vi "Start PJVS.vi"(6 "Requiested PJVS steps":u32, 7 "Requested PJVS frequency (Hz)":dbl, 8 "error in (pass through)":errorcluster, 10 "Maximal signal amplitude (V)":dbl, 11 "PJVS setup":T1={"PJVS type"=enum."AC-supraVOLTcontrol", "Status Refnum"=refnum, "AC-supraVOLTcontrol"={"IP address:port (0.0.0.0:0000)"="0.0.0.0:0000", "Timeouts"={"TCP Read & Write (ms)"=7000, "Sensors readout"=5000, "PJVS setup"=10000, "Nullmeter readout"=5000, "Multiplexer setup"=3000, "57XX setup"=15000, "Generator setup"=5000, "Synthesizer setup"=3000, "Sampler readout"=10000}, "Simulation mode"=FALSE, "Debug mode"=FALSE}, "NPL bias source"={"DataSocketCluster"={"Server Machine"="CZC", "Client Machine"="localhost", "Data"="P2", "TimeStamp"=0.0, "Count"=1, "Target Process"="General Server"}}, "Manual PJVS"={"PJVS frequency (Hz)"=0.0, "Reference voltages (V)"=[], "File with PJVS voltages"=path ""}, "VTT PJVS"={"some VTT only property"=""}} {"NPL bias source"."DataSocketCluster"."TimeStamp" format="%.2f"}) -> (0 "error out":errorcluster, 2 "PJVS reference voltages (1 period, V)":dbl[](array[numeric]), 3 "PJVS setup out":T1={"PJVS type"=enum."AC-supraVOLTcontrol", "Status Refnum"=refnum, "AC-supraVOLTcontrol"={"IP address:port (0.0.0.0:0000)"="0.0.0.0:0000", "Timeouts"={"TCP Read & Write (ms)"=7000, "Sensors readout"=5000, "PJVS setup"=10000, "Nullmeter readout"=5000, "Multiplexer setup"=3000, "57XX setup"=15000, "Generator setup"=5000, "Synthesizer setup"=3000, "Sampler readout"=10000}, "Simulation mode"=FALSE, "Debug mode"=FALSE}, "NPL bias source"={"DataSocketCluster"={"Server Machine"="CZC", "Client Machine"="localhost", "Data"="P2", "TimeStamp"=0.0, "Count"=1, "Target Process"="General Server"}}, "Manual PJVS"={"PJVS frequency (Hz)"=0.0, "Reference voltages (V)"=[], "File with PJVS voltages"=path ""}, "VTT PJVS"={"some VTT only property"=""}} {"NPL bias source"."DataSocketCluster"."TimeStamp" format="%.2f"}, 4 "Set PJVS steps":u32, 5 "Set frequency (Hz)":dbl)   [LabVIEW 2020]
doc: "Initialize the PJVS. Calls the initialization routine of the actual driver."
uses:
  Type definitions/PJVS.ctl
  Type definitions/PJVS Type.ctl
  external libraries/acsvcontrol-driver/Public/Type Definitions/Timeouts.ctl
  external libraries/JV modified NPL Bias source/DataSocketCluster external.ctl
  external libraries/acsvcontrol-driver/Public/Type Definitions/Waveform.ctl
  external libraries/acsvcontrol-driver/Public/Type Definitions/Multiplexer.ctl
  <vilib>/Utility/error.llb/Error Cluster From Error Code.vi
  <vilib>/ErrorRing/Error Ring.xnode
  external libraries/acsvcontrol-driver/ACSVcontrol-driver.lvlib
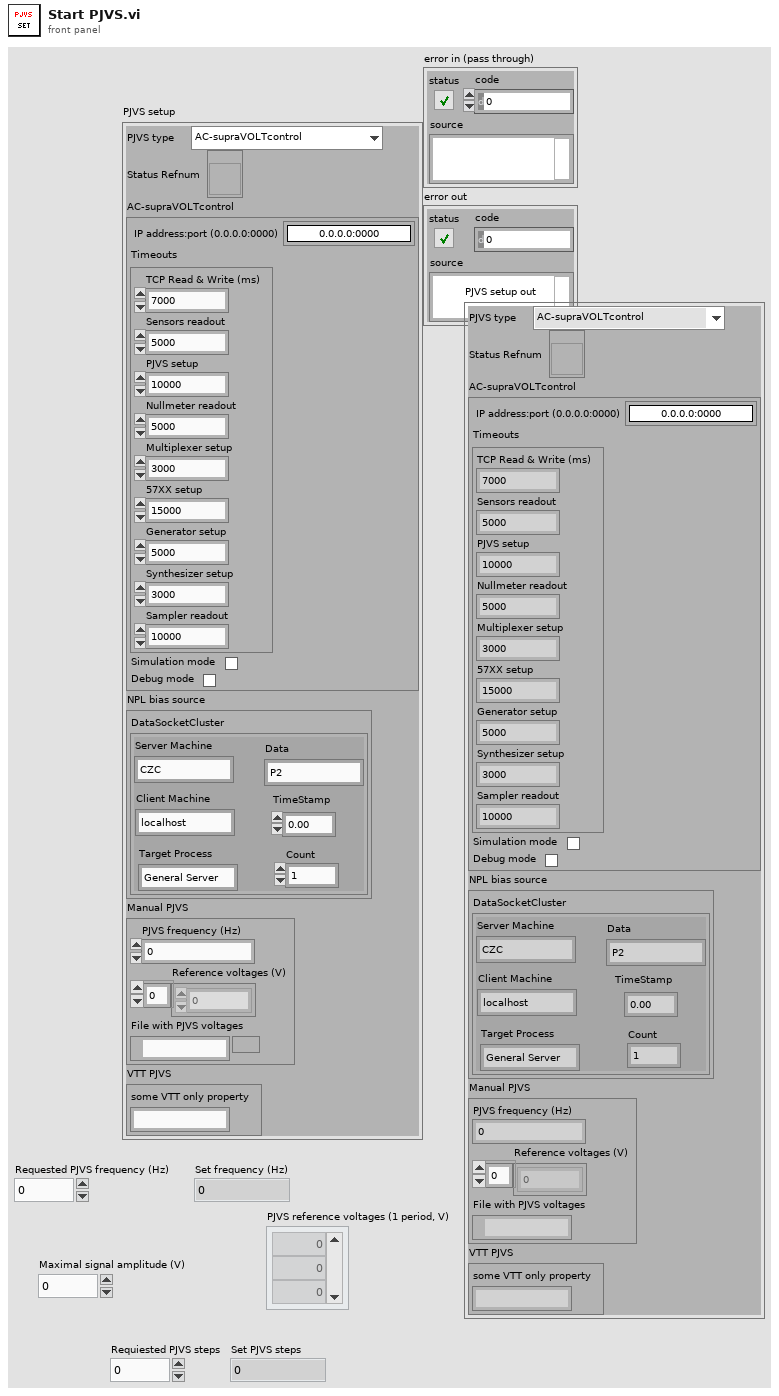
[diagram p1: front panel]
types:
  T1 = typedef "PJVS.ctl" = cluster{"PJVS type":T2, "Status Refnum":refnum<vi>, "AC-supraVOLTcontrol":cluster{"IP address:port (0.0.0.0:0000)":string, "Timeouts":T3, "Simulation mode":bool, "Debug mode":bool}, "NPL bias source":cluster{"DataSocketCluster":T4}, "Manual PJVS":cluster{"PJVS frequency (Hz)":dbl, "Reference voltages (V)":dbl[], "File with PJVS voltages":path}, "VTT PJVS":cluster{"some VTT only property":string}}
  T2 = typedef "PJVS Type.ctl" = enum16{"AC-supraVOLTcontrol", "JV modified NPL bias control", "Manual PJVS", "VTT PJVS"}
  T3 = typedef "ACSVcontrol-driver.lvlib/Timeouts.ctl" = cluster{"TCP Read & Write (ms)":i32, "Sensors readout":i32, "PJVS setup":i32, "Nullmeter readout":i32, "Multiplexer setup":i32, "57XX setup":i32, "Generator setup":i32, "Synthesizer setup":i32, "Sampler readout":i32}
  T4 = typedef "DataSocketCluster external.ctl" = cluster{"Server Machine":string, "Client Machine":string, "Data":string, "TimeStamp":dbl, "Count":i32, "Target Process":string}
  T5 = typedef "ACSVcontrol-driver.lvlib/Multiplexer.ctl" = enum16{"Short DC Nano / Voltmeter", "Short AC Sampler", "Short Switch DC (JVS->Nano)", "Short Switch AC (JVS->Digit)", "JVS-Voltmeter", "Channel A positive", "Channel A negative", "Channel B positive", "Channel B negative", "Channel C positive", "Channel C negative", "Nulldetector-Channel A+", "Nulldetector-Channel A-", "Nulldetector-Channel B+", "Nulldetector-Channel B-", "Nulldetector-Channel C+", "Nulldetector-Channel C-", "ext.Voltmeter-Channel A+", "ext.Voltmeter-Channel A-", "ext.Voltmeter-Channel B+", "ext.Voltmeter-Channel B-", "ext.Voltmeter-Channel C+", "ext.Voltmeter-Channel C-"}
  T6 = typedef "ACSVcontrol-driver.lvlib/Waveform.ctl" = enum16{"Sinewave", "Triangle", "Sawtooth", "Rectangle", "Arbitrary"}
  T7 = typedef "ACSVcontrol-driver.lvlib/PJVS Voltages.ctl" = cluster{"DC Voltage (S)":dbl, "AC Josephson Voltage RMS (V)":dbl, "Number of steps":i32, "AC Voltages (V)":dbl[]}
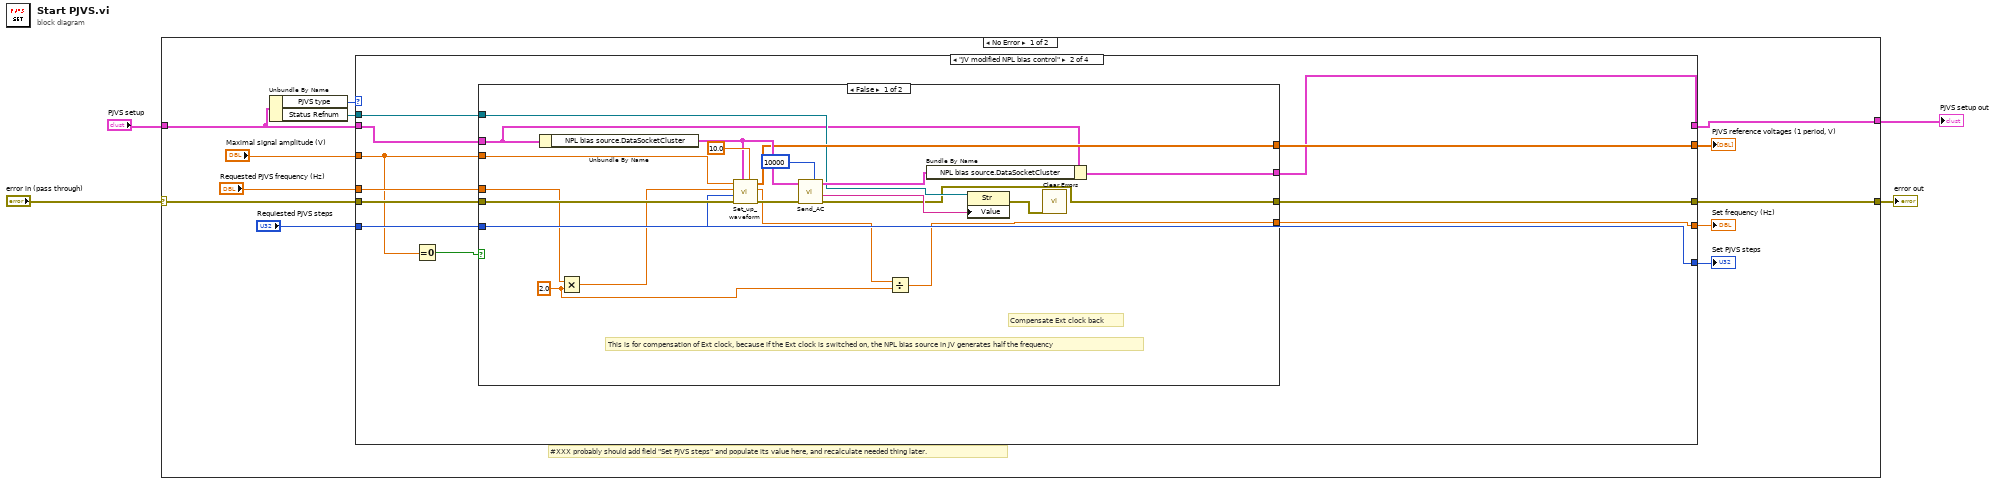
[diagram p0: block diagram]
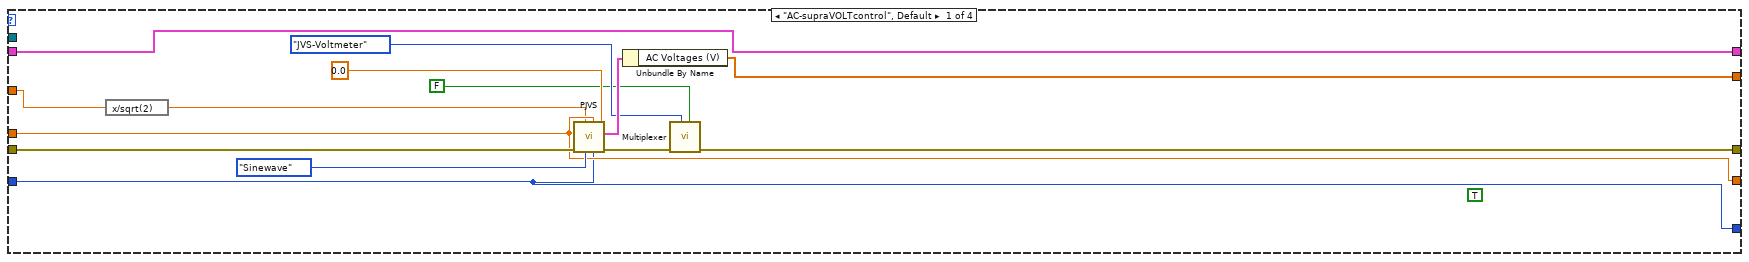
[diagram p2: hidden frame]
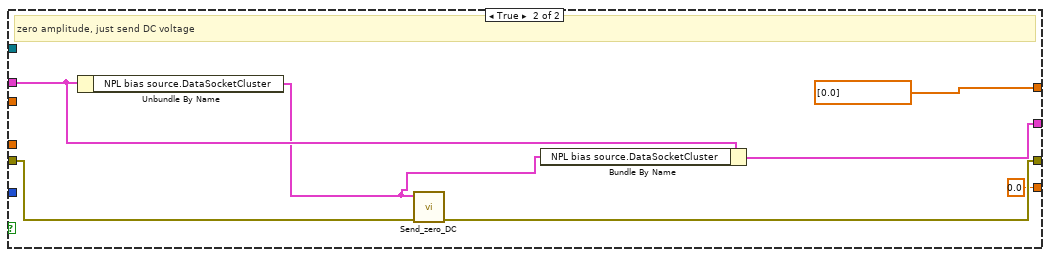
[diagram p3: hidden frame]
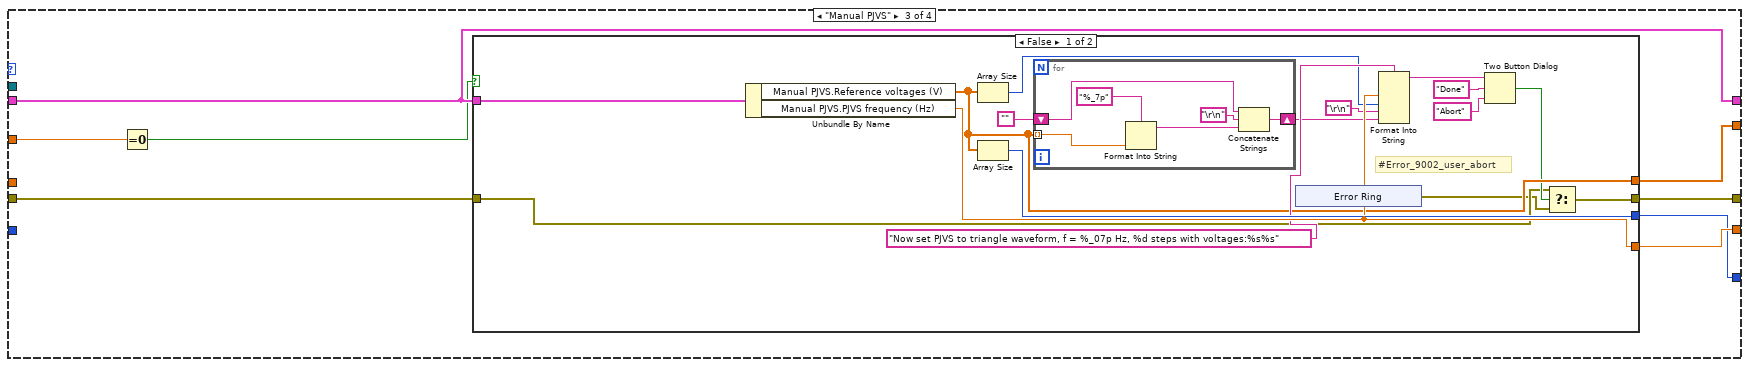
[diagram p4: hidden frame]
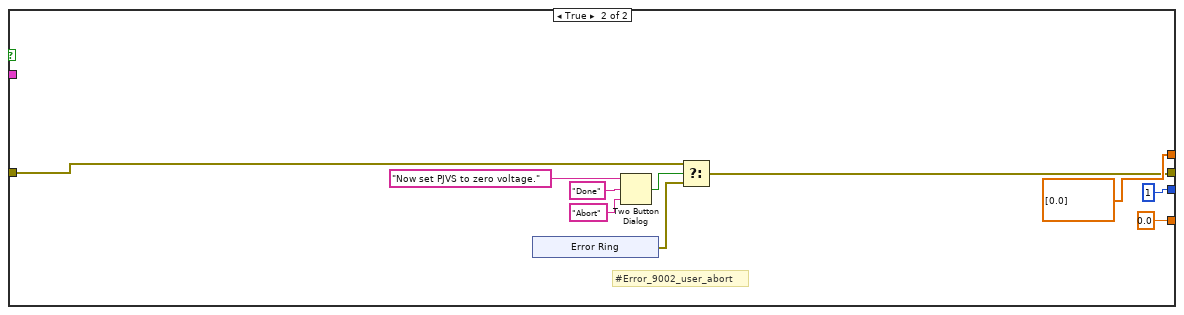
[diagram p5: hidden frame]
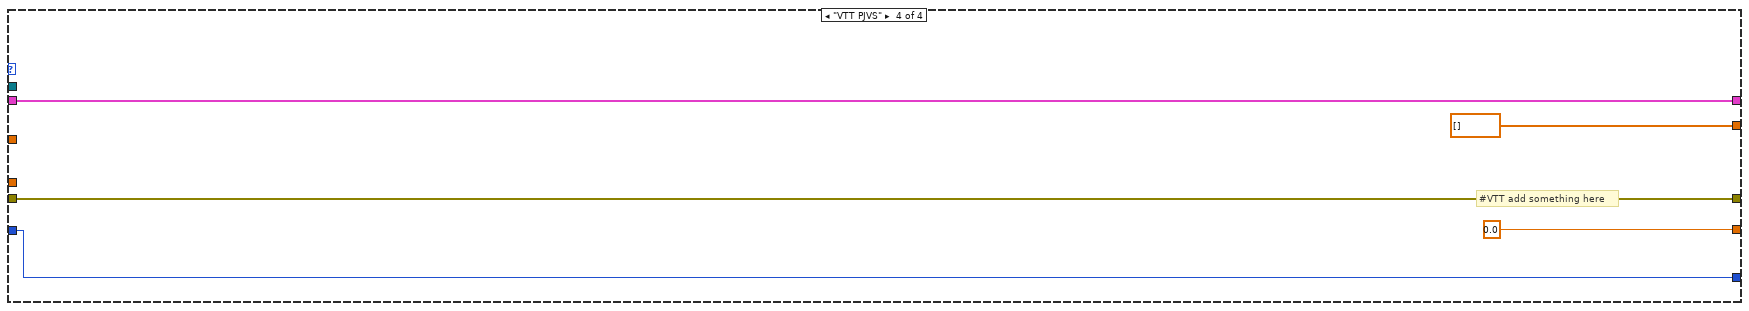
[diagram p6: hidden frame]
diagram:
  n1 = case shown="No Error" "error in (pass through)" {
    selector: "error in (pass through)" -> [w13 w125]
    tunnel: "PJVS setup" -> [w11 w124]
    tunnel: [w14 w125] -> w3
    tunnel: [w10 w124] -> w1
    frame No Error {
      # "#XXX probably should add field \"Set PJVS steps\" and populate its value here, and recalculate needed thing later."
      n2 = Unbundle By Name(w11) -> ("PJVS type"=w16:T2, "Status Refnum"=w15:refnum<vi>)
      n3 = case shown="\"JV modified NPL bias control\"" w16 {
        tunnel: w15 -> [_ w40 _ _]
        tunnel: w13 -> [w30 w39 w69 w122]
        tunnel: [w22 w38 w70 w122] -> w14
        tunnel: "Requested PJVS frequency (Hz)" -> [w21 w36 _ _]
        tunnel: "Maximal signal amplitude (V)" -> [w18 w34 w72 _]
        tunnel: "Requiested PJVS steps" -> [w19 w37 _ w119]
        tunnel: [w26 w41 w74 dbl[] [] ("Voltage at each step on PJVS curve")] -> w5
        tunnel: w11 -> [w20 w31 w76 w123]
        tunnel: [w21 w35 w75 0.0 ("Set frequency (Hz)")] -> w12
        tunnel: [w20 w32 w76 w123] -> w10
        tunnel: [w19 w37 w73 w119] -> w6
        frame "AC-supraVOLTcontrol", Default {
          (unwired) TRUE ("Waveform (F) (F:Sine, T:Square)")
          n4 = expression code="x/sqrt(2)"(w18) -> (w17:dbl)
          n5 = call "PJVS.vi"("Trim current (A) (+- 0.002)"=0.0, "Samples (2) (2 - 256)"=w19, "Frequency  (0 Hz) (0, 0.5 - 10e3)"=w21, "Waveform (Sinewave)"=Waveform."Sinewave", "Voltage (0 V DC/RMS) (DC: +- 10.1, AC: 0 - 7.2)"=w17, "error in (no error)"=w30) -> ("error out"=w25:errorcluster, "PJVS Voltages"=w27:T7)  [unwired: 4 in]
          n6 = Unbundle By Name(w27) -> ("AC Voltages (V)"=w26:dbl[])
          n7 = call "Multiplexer.vi"("AC (F) (F:Nano, T:Digitizer)"=FALSE, "Multiplexer (Short DC Nano / Voltmeter)"=Multiplexer."JVS-Voltmeter", "error in (no error)"=w25) -> ("error out"=w22:errorcluster)  [unwired: 8 in]
        }
        frame "JV modified NPL bias control" {
          n8 = Equal To 0?(x=w34) -> (x = 0?=w33:bool)
          n9 = case shown="False" w33 {
            tunnel: w34 -> [w59 _]
            tunnel: [w58 dbl[] [0.0] ("Voltage at each step on PJVS curve")] -> w41
            tunnel: w31 -> [w45 w68]
            tunnel: w40 -> [w55 _]
            tunnel: w39 -> [w53 w65]
            tunnel: [w43 w64] -> w38
            tunnel: w37 -> [w51 _]
            tunnel: w36 -> [w49 _]
            tunnel: [w46 0.0] -> w35
            tunnel: [w44 w67] -> w32
            frame False {
              w50 = 2.0 ("y")
              # "Compensate Ext clock back"
              # "This is for compensation of Ext clock, because if the Ext clock is switched on, the NPL bias source in JV generates half the frequency"
              n10 = Unbundle By Name(w45) -> ("NPL bias source.DataSocketCluster"=w60:T4)
              n11 = Multiply(x=w49, y=w50) -> (x*y=w48:dbl)
              n12 = call "Set_up_waveform.vi"("TimeOut Time (s)"=10.0, "DataSocketCluster In"=w60, "error in (no error)"=w53, "Steps on PJVS curve"=w51, "Frequency (Hz)"=w48, "Amplitude (V)"=w59) -> ("error IO"=w52:errorcluster, "Set frequency (Hz)"=w47:dbl, "Voltage at each step on PJVS curve"=w58:dbl[])  [unwired: 3 out]
              n13 = call "Send_AC.vi"("milliseconds to wait"=u32 10000, "error in (no error)"=w52, "DataSocketCluster In"=w60) -> ("error out"=w43:errorcluster, "Response to SEND AC"=w54:string, "DataSocketCluster out"=w56:T4)  [unwired: 6 in]
              n14 = Divide(x=w47, y=w50) -> (x/y=w46:dbl)
              n15 = Bundle By Name(cluster=w45, "NPL bias source.DataSocketCluster"=w56) -> (w44:T1)
              n16 = property class="Str"(reference=w55, "Value"=w54) -> (error out=w42:errorcluster)  [unwired: 1 in, 1 out]
              n17 = call <vilib>:"Clear Errors.vi"("error in (no error)"=w42) -> ()  [unwired: 5 in, 2 out]
            }
            frame True {
              # "zero amplitude, just send DC voltage"
              n18 = Unbundle By Name(w68) -> ("NPL bias source.DataSocketCluster"=w66:T4)
              n19 = call "Send_zero_DC.vi"("error in (no error)"=w65, "machine"=w66) -> ("error out"=w64:errorcluster)  [unwired: 8 in, 1 out]
              n20 = Bundle By Name(cluster=w68, "NPL bias source.DataSocketCluster"=w66) -> (w67:T1)
            }
          }
        }
        frame "Manual PJVS" {
          n21 = Equal To 0?(x=w72) -> (x = 0?=w71:bool)
          n22 = case shown="False" w71 {
            tunnel: w76 -> [w92 _]
            tunnel: [w90 0.0 ("PJVS frequency (Hz)")] -> w75
            tunnel: [w86 dbl[] [0.0] ("Reference voltages (V)")] -> w74
            tunnel: [w91 1] -> w73
            tunnel: w69 -> [w79 w106]
            tunnel: [w78 w105] -> w70
            frame False {
              # "#Error_9002_user_abort"
              n23 = Unbundle By Name(w92) -> ("Manual PJVS.Reference voltages (V)"=w86:dbl[], "Manual PJVS.PJVS frequency (Hz)"=w90:dbl)
              n24 = Array Size(array=w86) -> (size(s)=w85:i32)
              n25 = Array Size(array=w86) -> (size(s)=w91:i32)
              n26 = for {
                tunnel: w86 -> [w103] mode=indexing
                shift-right: [w98] -> w83
                shift-left: "" -> [w99]
                n27 = Format Into String(format string="%_7p", w103) -> (resulting string=w101:string)  [unwired: 2 in, 1 out]
                n28 = Concatenate Strings(w99, "\r\n", w101) -> (w98:string)
              }
              n29 = xnode "Error Ring"() -> ("error out"=w77:errorcluster)
              n30 = Format Into String(format string="Now set PJVS to triangle waveform, f = %_07p Hz, %d steps with voltages:%s%s" ("message"), w90, w85, "\r\n", w83) -> (resulting string=w88:string)  [unwired: 2 in, 1 out]
              n31 = Two Button Dialog(message=w88, 1:"Abort" ("F button name (\"Cancel\")"), 2:"Done" ("T button name (\"OK\")")) -> (T button?=w80:bool)
              n32 = Select(t=w79, s=w80, f=w77) -> (s? t:f=w78:errorcluster)
            }
            frame True {
              # "#Error_9002_user_abort"
              n33 = xnode "Error Ring"() -> ("error out"=w104:errorcluster)
              n34 = Two Button Dialog(message="Now set PJVS to zero voltage.", 1:"Abort" ("F button name (\"Cancel\")"), 2:"Done" ("T button name (\"OK\")")) -> (T button?=w107:bool)
              n35 = Select(t=w106, s=w107, f=w104) -> (s? t:f=w105:errorcluster)
            }
          }
        }
        frame "VTT PJVS" {
          # "#VTT add something here"
        }
      }
      "Set PJVS steps" <- w6
      "Set frequency (Hz)" <- w12
      "PJVS reference voltages (1 period, V)" <- w5
    }
    frame Error {
    }
  }
  "error out" <- w3
  "PJVS setup out" <- w1
